vi "P1.vi"() -> ()   [LabVIEW 2025]
uses:
  <vilib>/Utility/file.llb/Write Delimited Spreadsheet (DBL).vi
panel:
  out "Waveform Chart":dynamicdata(graph)
  out "Data":dbl
  in  "stop 2":bool
  in  "Voltaje":dbl(slide) scale=0.0..5.0
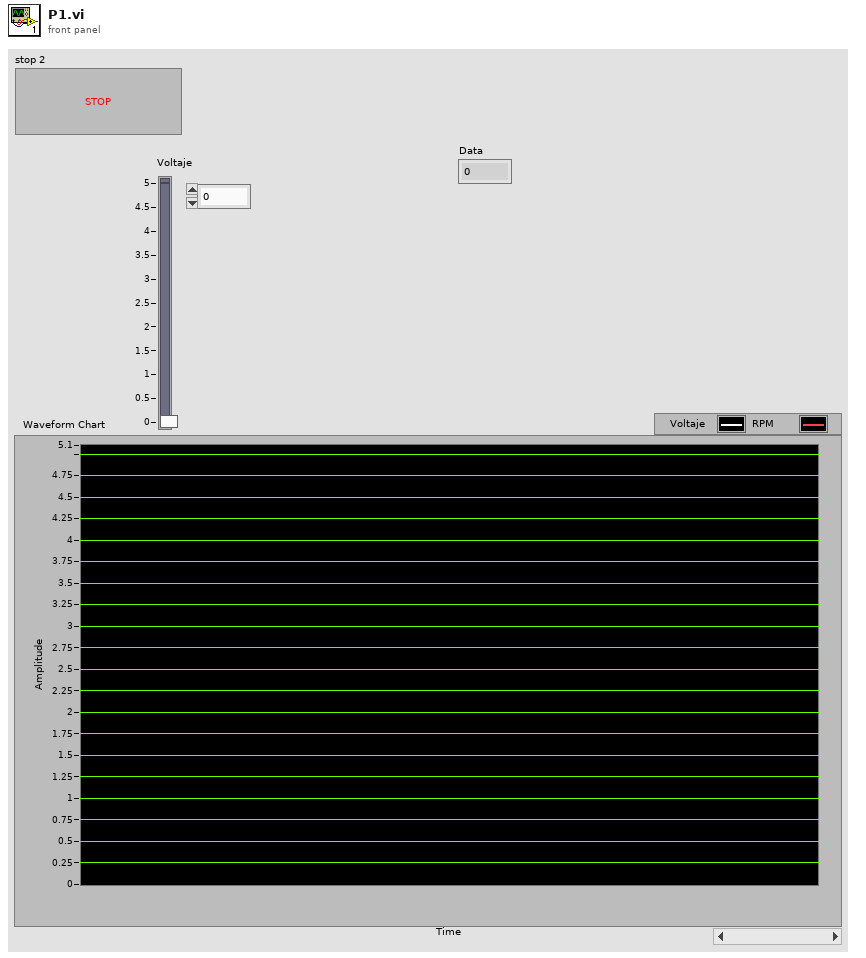
[diagram p1: front panel]
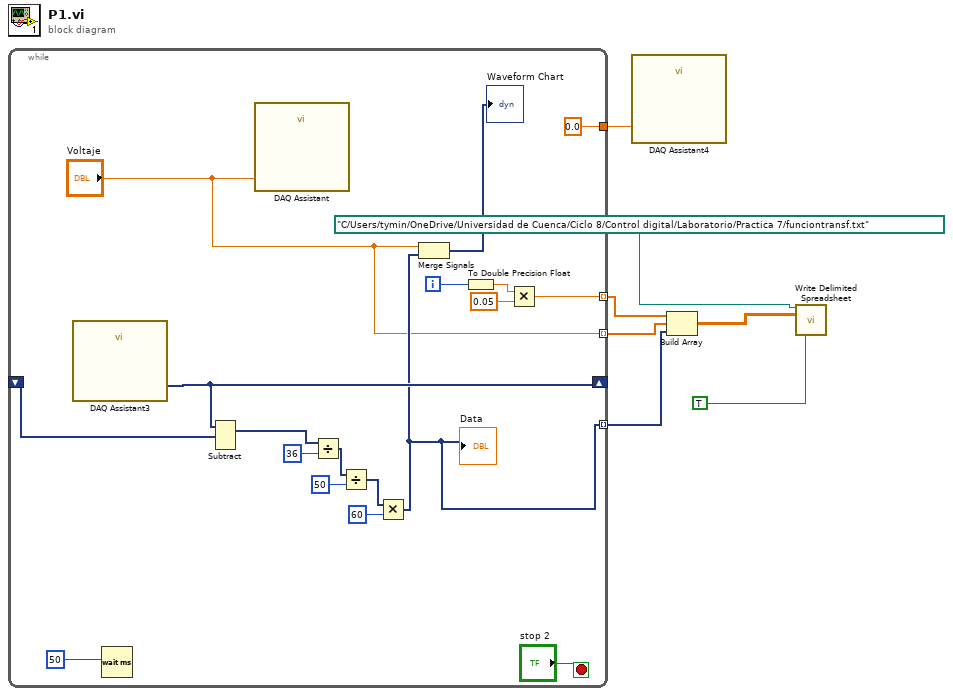
[diagram p0: block diagram]
diagram:
  n1 = while {
    shift-right: [w15] -> _
    shift-left: _ -> [w23]
    tunnel: [w14] -> w5 mode=indexing
    tunnel: [w10] -> w7 mode=indexing
    tunnel: ["Voltaje"] -> w6 mode=indexing
    tunnel: [0.0 ("data")] -> w1
    i -> [w11]
    stop <- "stop 2" stop-if-true
    n2 = call "DAQ Assistant3"() -> ("data"=w15:dynamicdata)  [unwired: 16 in, 3 out]
    n3 = Wait (ms)(milliseconds to wait=u32 50 ("millisecond timer value")) -> ()  [unwired: 1 out]
    n4 = Subtract(1:w23, 2:w15) -> (0:w22:dynamicdata)  [unwired: 1 in, 1 out]
    n5 = call "DAQ Assistant"("data"="Voltaje") -> ()  [unwired: 17 in, 2 out]
    n6 = Divide(x=w22, y=36) -> (x/y=w17:dynamicdata)
    n7 = Divide(x=w17, y=50) -> (x/y=w18:dynamicdata)
    n8 = Multiply(x=w18, y=60) -> (x*y=w14:dynamicdata)
    "Data" <- w14
    n9 = Merge Signals("Voltaje", w14) -> (→"Waveform Chart":dynamicdata)
    n10 = To Double Precision Float(number=w11) -> (double precision float=w12:dbl)
    n11 = Multiply(x=w12, y=0.05) -> (x*y=w10:dbl)
  }
  n12 = call "DAQ Assistant4"("data"=w1) -> ()  [unwired: 17 in, 2 out]
  n13 = Build Array(w7, w6, w5) -> (w4:dbl[][])
  n14 = call-poly <vilib>:"Write Delimited Spreadsheet.vi"("file path (dialog if empty)"=path "C:/Users/tymin/OneDrive/Universidad de Cuenca/Ciclo 8/Control digital/Laboratorio/Practica 7/funciontransf.txt", "2D data"=w4, "transpose? (no:F)"=TRUE) -> ()  [unwired: 11 in, 2 out]
